vi "RVC Rotation about a Vector.vi"() -> ()   [LabVIEW 2013]
uses:
  <vilib>/Analysis/Matrix/Datatypes/ComplexMatrix.ctl
  <vilib>/Analysis/_algsub.llb/Vector Norm.vi
  <vilib>/Analysis/_algsub.llb/Real Vector Norm.vi
  <vilib>/Analysis/baseanly.llb/Outer Product.vi
  <vilib>/Analysis/baseanly.llb/Real Outer Product.vi
  <vilib>/robotics/Kinematics/Create Lie Group Matrix.vi
  <vilib>/Analysis/7linalg.llb/Real Eigenvalues and Vectors.vi
  <vilib>/Analysis/7linalg.llb/Create Special Matrix.vi
  <vilib>/Analysis/7linalg.llb/Create Special Real Matrix.vi
  <vilib>/Analysis/Matrix/Numeric/Multiply/Multiply.vi
  <vilib>/Analysis/Matrix/Numeric/Multiply/Multiply - RM,R.vi
  <vilib>/Analysis/Matrix/Numeric/Multiply/Multiply - R,RM.vi
  <vilib>/Analysis/Matrix/Numeric/Add/Add.vi
  <vilib>/Analysis/Matrix/Numeric/Add/Add - RM,RM.vi
  <vilib>/robotics/Kinematics/NI_Kinematics.lvlib
  <vilib>/Analysis/NI_AALPro.lvlib
  <vilib>/Analysis/Matrix/NI_Matrix.lvlib
panel:
  out "RPY transformation":picture
  out "transformation matrix":picture
  out "Eigenvectors":T1
  out "Eigenvalues":cdb[](array[numeric])
  out "vector":dbl[](array[numeric])
  out "theta":dbl
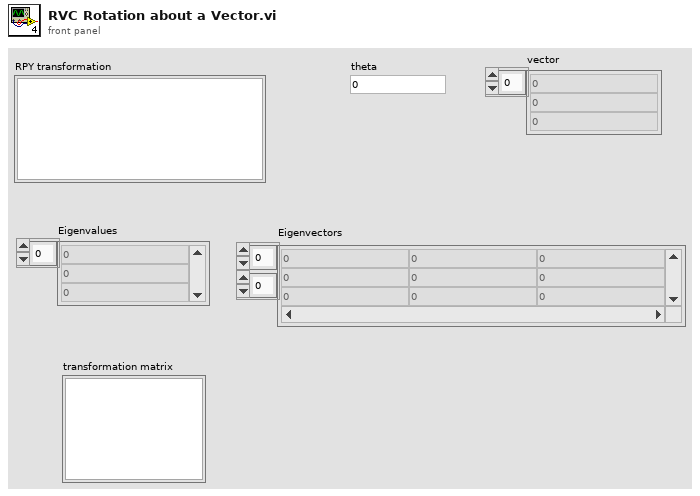
[diagram p1: front panel]
types:
  T1 = typedef "NI_Matrix.lvlib/ComplexMatrix.ctl" = cdb[][]
  T2 = typedef "NI_Matrix.lvlib/RealMatrix.ctl" = dbl[][]
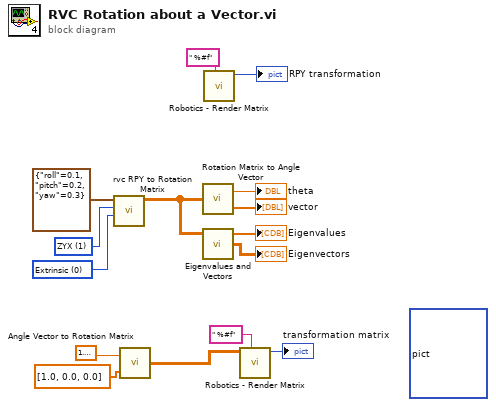
[diagram p0: block diagram]
diagram:
  (unwired) picture bytes[498] ("transformation matrix")
  w4 = u16 1 items=["XYZ", "ZYX"] ("Convension")
  w3 = u16 0 items=["Extrinsic", "Intrinsic"] ("type of rotations")
  n1 = call "rvc RPY to Rotation Matrix.vi"("type of rotations"=w3, "Convension"=w4, "angles"=cluster{"roll":dbl, "pitch":dbl, "yaw":dbl} {"roll"=0.1, "pitch"=0.2, "yaw"=0.3}) -> ("rotation matrix"=w1:T2)  [unwired: 8 in]
  n2 = call <vilib>:"Angle Vector to Rotation Matrix.vi"("vector"=dbl[] [1.0, 0.0, 0.0], "angle"=1.5707963267948966) -> ("rotation matrix"=w8:T2)
  n3 = call <vilib>:"Rotation Matrix to Angle Vector.vi"("rotation matrix"=w1) -> ("angle"=→"theta":dbl, "vector"=→"vector":dbl[])
  n4 = call-poly <vilib>:"Eigenvalues and Vectors.vi"("Input Matrix"=w1) -> ("Eigenvectors"=→"Eigenvectors":T1, "Eigenvalues"=→"Eigenvalues":cdb[])  [unwired: 2 in, 1 out]
  n5 = call "Robotics - Render Matrix.vi"("format string"=" %#f") -> ("picture out"=→"RPY transformation":picture)  [unwired: 10 in]
  n6 = call "Robotics - Render Matrix.vi"("format string"=" %#f", "A"=w8) -> ("picture out"=→"transformation matrix":picture)  [unwired: 9 in]
